vi "IDN.vi"(7 "byte count (60)":u32=60, 8 "error in (no error)":errorcluster, 11 "Reference in":T1={"Device"="", "Function"="", "delay"=20}) -> (0 "error out":errorcluster, 2 "answer":string, 3 "Reference out":T1={"Device"="", "Function"="", "delay"=20})   [LabVIEW 2021, in "Rigol DM3052.lvlib"]
uses:
  Rigol DM3052.lvlib
  Reference.ctl
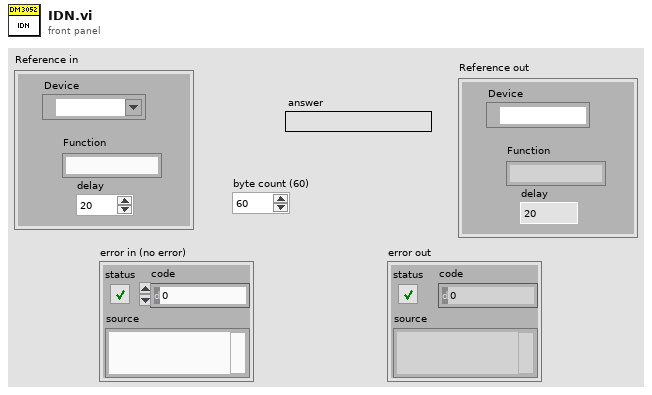
[diagram p1: front panel]
types:
  T1 = typedef "Rigol DM3052.lvlib/Reference.ctl" = cluster{"Device":refnum<visa-resource-name>, "Function":string, "delay":u32}
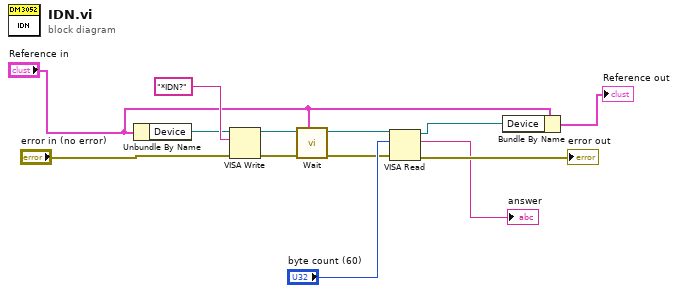
[diagram p0: block diagram]
diagram:
  n1 = Unbundle By Name("Reference in") -> ("Device"=w8:refnum<visa-resource-name>)
  n2 = VISA Write(VISA resource name=w8, write buffer="*IDN?", error in (no error)="error in (no error)") -> (VISA resource name out=w7:refnum<visa-resource-name>, error out=w6:errorcluster)  [unwired: 1 out]
  n3 = call "Wait.vi"("Reference in"="Reference in", "error in (no error)"=w6, "Device in"=w7) -> ("error out"=w5:errorcluster, "Device out"=w4:refnum<visa-resource-name>)  [unwired: 7 in]
  n4 = VISA Read(VISA resource name=w4, byte count="byte count (60)", error in (no error)=w5) -> (VISA resource name out=w2:refnum<visa-resource-name>, read buffer=→"answer":string, error out=→"error out":errorcluster)  [unwired: 1 out]
  n5 = Bundle By Name(cluster="Reference in", "Device"=w2) -> (→"Reference out":T1)
